vi "daniel tinkering with vision.vi"() -> ()   [LabVIEW 2013]
uses:
  <vilib>/Rock Robotics/WPI/Camera/WPI_CameraSettings Read MJPG.ctl
  <vilib>/Rock Robotics/WPI/Camera/WPI_CameraImageSize.ctl
  <vilib>/vision/NI_Vision_Development_Module.lvlib
panel:
  out "Image":T1(plugin-control)
  in  "Red Range":cluster{"Lower value":i32, "Upper value":i32}={"Lower value"=0, "Upper value"=255}
  in  "Green Range":cluster{"Lower value":i32, "Upper value":i32}={"Lower value"=0, "Upper value"=255}
  in  "Blue Range":cluster{"Lower value":i32, "Upper value":i32}={"Lower value"=0, "Upper value"=255}
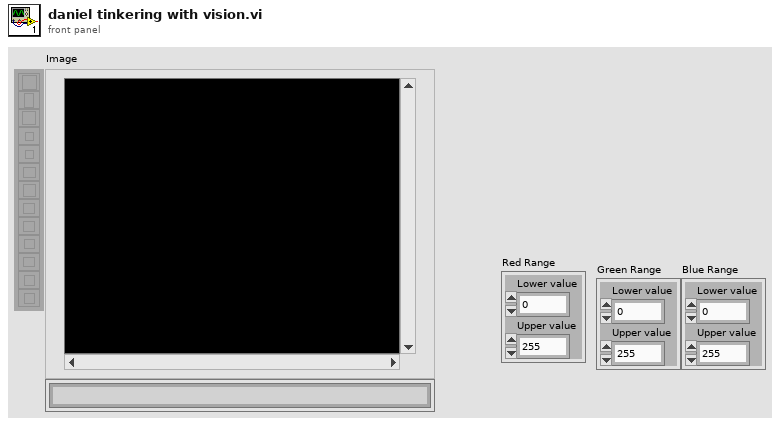
[diagram p1: front panel]
types:
  T1 = typedef "IMAQ Image.ctl" = refnum<image>
  T2 = typedef "WPI_CameraSettings Read MJPG.ctl" = cluster{"fps":i32, "compression":i32, "Image Size":T3}
  T3 = typedef "WPI_CameraImageSize.ctl" = enum16{"640x480", "320x240", "160x120"}
  T4 = enum32{"Gray", "Binary", "Gradient", "Rainbow", "Temperature"}
  T5 = typedef "Particle Parameters" = i32
  T6 = cluster{"Measurement Parameter":T5, "Range Lower Value":dbl, "Range Upper Value":dbl, "Range":bool, "Measurement Type":bool}[]
  T7 = typedef "Image Type" = u32
  T8 = cluster{"Area":dbl, "Number of Holes":dbl, "Bounding Rect":cluster{"Left":dbl, "Top":dbl, "Right":dbl, "Bottom":dbl}, "Center of Mass":cluster{"X":dbl, "Y":dbl}, "Orientation":dbl, "Dimensions":cluster{"Width":dbl, "Height":dbl}}[]
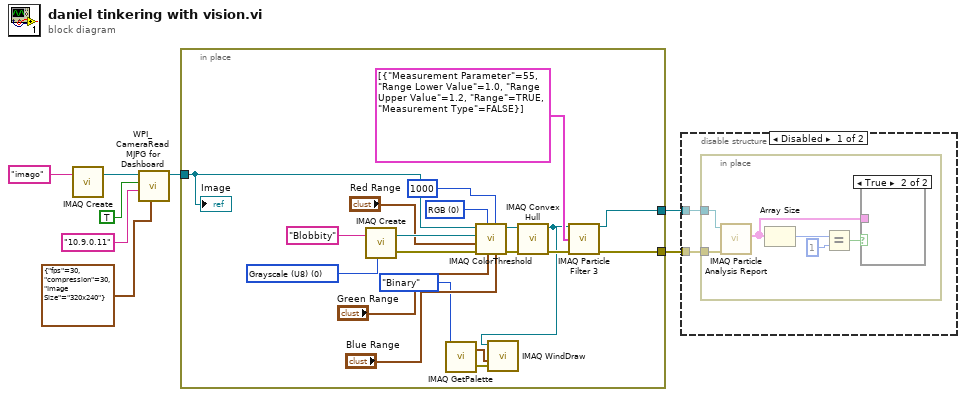
[diagram p0: block diagram]
diagram:
  n1 = call "IMAQ Create"("Image Name"="imago") -> ("New Image"=w5:T1)  [unwired: 4 in, 1 out]
  n2 = call <vilib>:"WPI_CameraRead MJPG for Dashboard.vi"("Camera Settings"=T2 {"fps"=30, "compression"=30, "Image Size"=enum."320x240"}, "Camera IP"="10.9.0.11", "Enable"=TRUE, "Refnum in"=w5) -> ("Refnum out"=w3:T1)  [unwired: 4 in, 3 out]
  n3 = in-place {
    in-place-border: w3 -> [w16]
    in-place-border: [w10] -> w8
    in-place-border: [w17] -> w7
    w22 = u16 0 items=["RGB", "HSL", "HSV", "HSI"] ("Color Mode")
    w27 = T7 0 items=["Grayscale (U8)", "Grayscale (I16)", "Grayscale (SGL)", "Complex (CSG)", "RGB (U32)", "HSL (U32)", "RGB (U64)", "Grayscale (U16)"] ("Image Type")
    n4 = call "IMAQ Create"("Image Name"="Blobbity", "Image Type"=w27) -> ("New Image"=w26:T1, "error out"=w19:errorcluster)  [unwired: 3 in]
    n5 = call "IMAQ GetPalette"("Palette Number (gray)"=T4."Binary") -> ("Color Palette"=w13:cluster{"Red":u8, "Green":u8, "Blue":u8}[], "error out"=w12:errorcluster)  [unwired: 4 in]
    n6 = call "IMAQ ColorThreshold"("Blue or Luma or Val or Inten Range"="Blue Range", "Replace Value"=1000, "Green or Sat Range"="Green Range", "Color Mode"=w22, "error in (no error)"=w19, "Red or Hue Range"="Red Range", "Image Dst"=w26, "Image Src"=w16) -> ("error out"=w20:errorcluster, "Image Dst Out"=w14:T1)  [unwired: 2 in]
    n7 = call "IMAQ Convex Hull"("error in (no error)"=w20, "Image Src"=w14) -> ("error out"=w18:errorcluster, "Image Dst Out"=w9:T1)  [unwired: 8 in]
    n8 = call "IMAQ WindDraw"("error in (no error)"=w12, "Color Palette"=w13, "Image"=w9) -> ()  [unwired: 7 in, 2 out]
    n9 = call "IMAQ Particle Filter 3"("Image Src"=w9, "Selection Values"=T6 [{"Measurement Parameter"=55, "Range Lower Value"=1.0, "Range Upper Value"=1.2, "Range"=TRUE, "Measurement Type"=FALSE}], "error in (no error)"=w18) -> ("Image Dst Out"=w10:T1, "error out"=w17:errorcluster)  [unwired: 10 in, 1 out]
    "Image" <- w16
  }
  n10 = disable-structure shown="Disabled" {
    disable-tunnel: w8 -> [w30 _]
    disable-tunnel: w7 -> [w29 _]
    frame Disabled {
      n11 = in-place {
        in-place-border: w30 -> [w36]
        in-place-border: w29 -> [w35]
        n12 = call "IMAQ Particle Analysis Report"("error in (no error)"=w35, "Image"=w36) -> ("Particle Reports (Pixels)"=w31:T8)  [unwired: 4 in, 5 out]
        n13 = Array Size(array=w31) -> (size(s)=w34:i32)
        n14 = Equal?(x=w34, y=1) -> (x = y?=w32:bool)
        n15 = case shown="True" w32 {
          tunnel: w31 -> [_ _]
          frame False {
          }
          frame True {
          }
        }
      }
    }
    frame Enabled {
    }
  }
